vi "2_VisualizeModulePositioning2.vi"(0 "Placement Monitor":T6(plugin-control), 1 "Calibrated positions of fiducials [mm]":dbl[][](array[numeric])=[[-675.4228165149058, -196.82430550413875, -11.55], [-579.8428201474238, -196.8506568257386, -11.55], [-579.816468825824, -101.27066045825673, -11.55], [-675.3964651933059, -101.24430913665685, -11.55], [-577.422820239396, -196.8513240176017, -11.55], [-481.84282387191405, -196.87767533920157, -11.55], [-481.8164725503142, -101.29767897171968, -11.55], [-577.396468917796, -101.2713276501198, -11.55], [-479.42282396388623, -196.87834253106465, -11.55], [-383.8428275964043, -196.90469385266454, -11.55], [-383.81647627480436, -101.32469748518264, -11.55], [-479.3964726422863, -101.29834616358275, -11.55], [-381.42282768837646, -196.90536104452758, -11.55], [-285.8428313208945, -196.93171236612747, -11.55], [-285.8164799992946, -101.35171599864559, -11.55], [-381.39647636677654, -101.3253646770457, -11.55], [-283.4228314128667, -196.93237955799054, -11.55], [-187.84283504538473, -196.95873087959043, -11.55], [-187.8164837237848, -101.37873451210854, -11.55], [-283.39648009126677, -101.35238319050865, -11.55], [-185.42283513735697, -196.9593980714535, -11.55], [-89.84283876987502, -196.98574939305337, -11.55], [-89.81648744827521, -101.40575302557149, -11.55], [-185.39648381575705, -101.3794017039716, -11.55], [-87.42283886184703, -196.98641658491644, -11.55], [8.157157505634814, -197.01276790651633, -11.55], [8.183508827234618, -101.43277153903443, -11.55], [-87.39648754024722, -101.40642021743454, -11.55], [10.57715741366269, -197.01343509837938, -11.55], [106.15715378114453, -197.0397864199793, -11.55], [106.18350510274433, -101.45979005249738, -11.55], [10.603508735262494, -101.4334387308975, -11.55], [108.57715368917252, -197.04045361184234, -11.55], [204.15715005665436, -197.06680493344223, -11.55], [204.18350137825416, -101.48680856596033, -11.55], [108.60350501077232, -101.46045724436046, -11.55], [206.57714996468223, -197.0674721253053, -11.55], [302.1571463321641, -197.09382344690516, -11.55], [302.1834976537639, -101.5138270794233, -11.55], [206.60350128628204, -101.4874757578234, -11.55], [304.57714624019206, -197.09449063876826, -11.55], [400.1571426076739, -197.12084196036813, -11.55], [400.1834939292737, -101.54084559288623, -11.55], [304.60349756179187, -101.51449427128635, -11.55], [402.5771425157018, -197.1215091522312, -11.55], [498.15713888318373, -197.1478604738311, -11.55], [498.18349020478354, -101.56786410634919, -11.55], [402.6034938373016, -101.5415127847493, -11.55], [500.5771387912116, -197.14852766569413, -11.55], [596.1571351586933, -197.17487898729405, -11.55], [596.1834864802931, -101.59488261981214, -11.55], [500.6034901128114, -101.56853129821225, -11.55]], 2 "XYZ .NET Refnum in":refnum<k24>, 3 "Axis Speeds":T10={"X [mm/s]"=25.0, "Y [mm/s]"=25.0, "Z [mm/s]"=25.0}, 4 "Module fiducial marker":T7, 5 "N modules":i32=13, 6 "Sensor Pattern":T8(ring)=enum."ATLAS12", 7 "error in (no error)":errorcluster, 8 "Templates path":path=path "C:/Users/Aerotech/Documents/BNL_ThermomechanicalStave", 9 "Calibration [um/pix]":dbl=1.58, 10 "Current Build Phase":refnum<vi>, 12 "Module #":refnum<vi>, 13 "Placement tolerance [um]":dbl=25.0, 14 "Tape Type":T4=enum."Left stereo", 16 "Module Report":refnum<vi>, 17 "Base notes":string, 18 "Reports path":path=path "C:/Users/Aerotech/cernbox/BNL/Stave Assembly Records/2017-05-10") -> (22 "XYZ .NET Refnum out":refnum<k24>, 27 "error out":errorcluster)   [LabVIEW 2016]
uses:
  Utils/Enum_TypeDefinitions/Enum_TypeDef_FidMarkers.ctl
  C:/Users/Aerotech/Documents/BNL_ThermomechanicalStave/AerotechLibraries/Bin/Aerotech.A3200.dll
  AerotechLibraries/Bin/Aerotech.A3200.dll
  Utils/Enum_TypeDefinitions/Enum_TypeDef_CornerSelection.ctl
  Utils/Enum_TypeDefinitions/Enum_TypeDef_TapeType.ctl
panel:
  in  "Exit Module Placement":bool
  in  "Exit to survey or glue":bool
  out "Current task:":string
  in  "Tab Control: Positioning and Surveys":T1(tab)
  out "Offset interpreter":T2
  in  "User Report: Current Module":T3
  out "X offset [um]":sgl
  out "Y offset [um]":sgl
  in  "Module corner loop stop":bool
  in  "User notes":string="Type your note here...."
  out "Module # str":string
  in  "Assembly step":string(combo)
  in  "Calibrate distance?":bool=TRUE
  in  "Send XYZ stage beyond EOS":bool
  in  "Work on Corner...":T5=enum."[Exit]"
  in  "Work on Module #...":i32
  in  "Tab Control":enum32{"Fiducial marker", "Error reporting"}(tab)
  out "Fiducial Template":T6(plugin-control)
  out "Mark string":string
  out "Current Stage Position":T9
  out "Module Progress Report":T11(array[cluster])
  # "VISUALIZE MODULE PLACEMENT Brandeis University - Brookhaven National Laboratory * ATLAS Phase II Inner Tracker Upgrade"
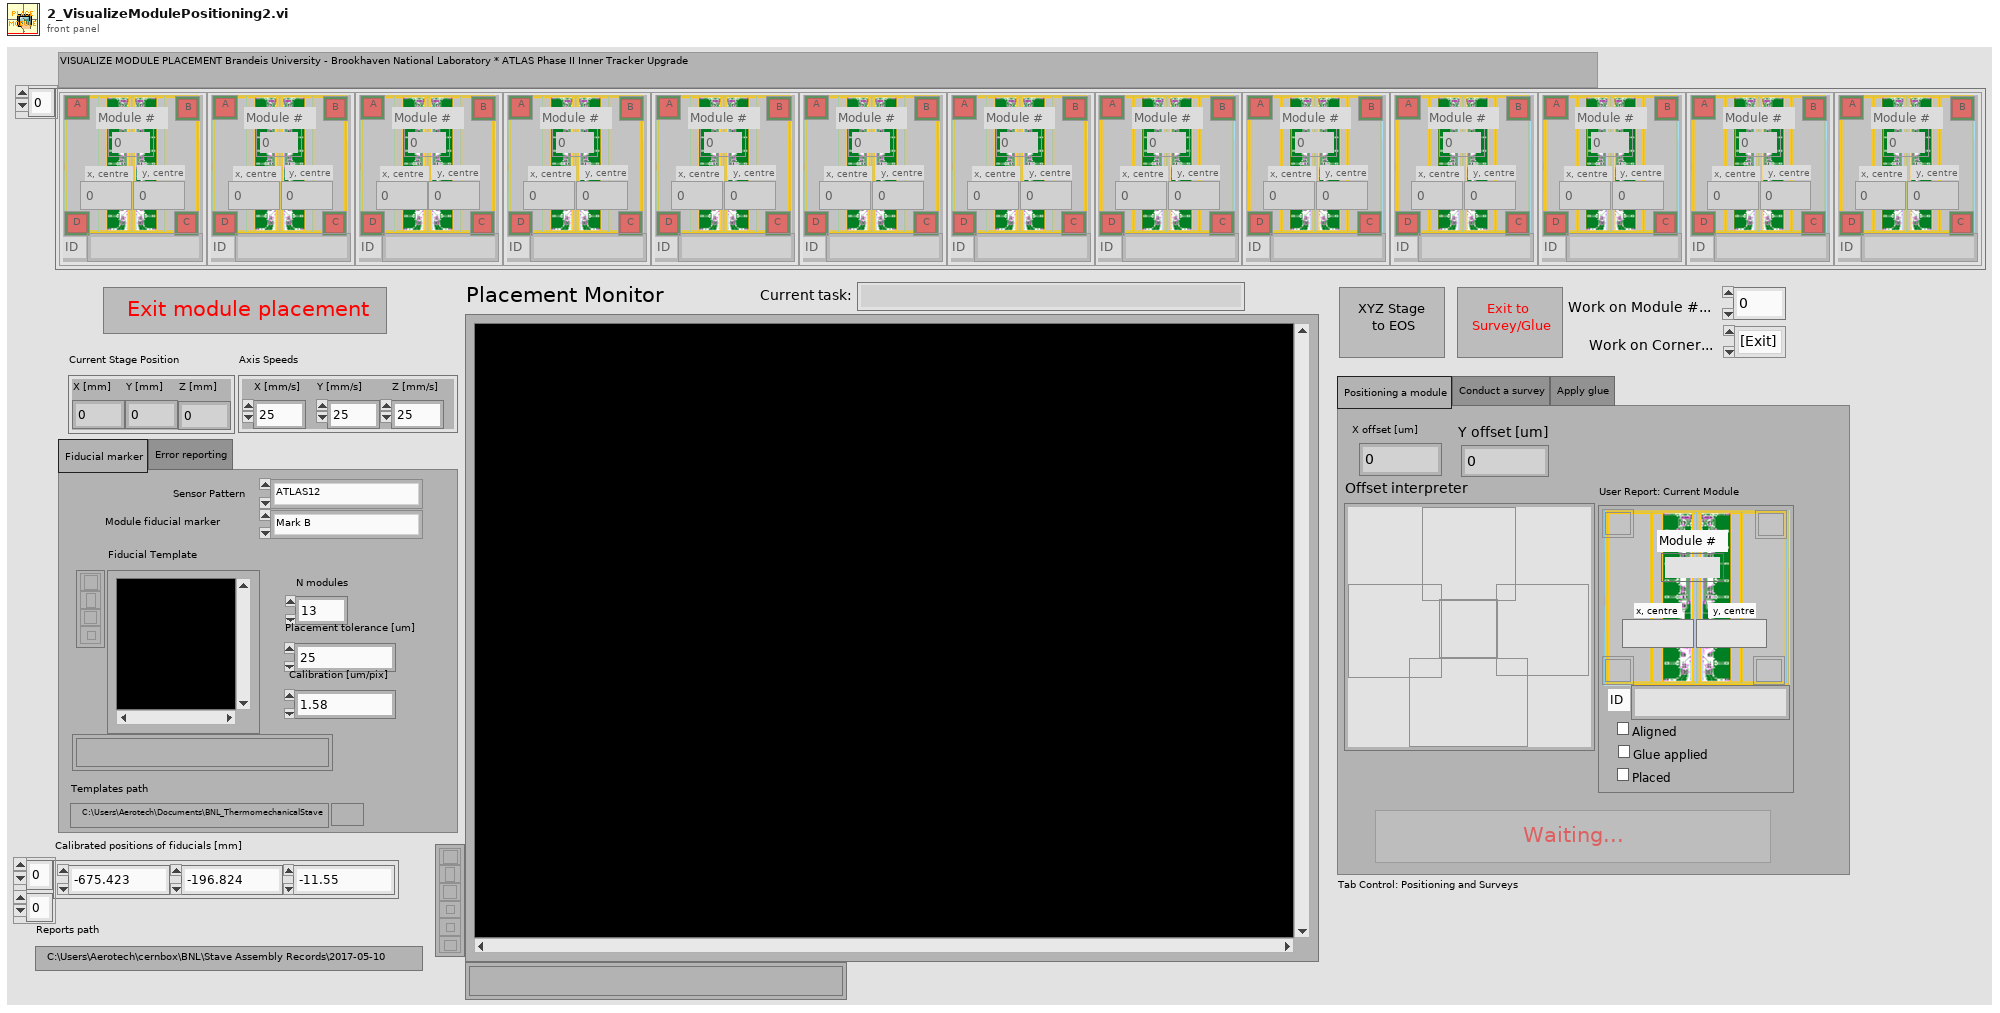
[diagram p1: front panel]
types:
  T1 = enum32{"Positioning a module", "Conduct a survey", "Apply glue"}
  T2 = cluster{"Offset Interpreter - Right":bool, "Offset Interpreter - forward":bool, "Offset Interpreter - backward":bool, "Offset Interpreter - Left":bool, "Placement Confirmation":bool}
  T3 = cluster{"B":bool, "A":bool, "D":bool, "C":bool, "ID":string, "Module #":i32, "x, centre":dbl, "y, centre":dbl, "Aligned":bool, "Glue applied":bool, "Placed":bool}
  T4 = typedef "Enum_TypeDef_TapeType.ctl" = enum16{"Right stereo", "Left stereo", "Stereo (Sutcliffe NP49-01-100 01-Mar-16)", "Axial (Sutcliffe NP49-01-100 01-Mar-16)"}
  T5 = typedef "Enum_TypeDef_CornerSelection.ctl" = enum16{"A", "B", "C", "D", "[Exit]"}
  T6 = typedef "IMAQ Image.ctl" = refnum<image>
  T7 = typedef "Enum_TypeDef_FidMarkers.ctl" = enum16{"Mark B", "Mark C", "Strip Corner", "Mark I (Slim/17)", "Mark E (Slim/17)", "Mark F (Slim/17)", "Mark G (Slim/17)", "Mark A (12)", "KaptonSpacers"}
  T8 = enum16{"ATLAS07", "ATLAS12", "ATLAS12Slim", "ATLAS17LS"}
  T9 = cluster{"X [mm]":dbl, "Y [mm]":dbl, "Z [mm]":dbl}
  T10 = cluster{"X [mm/s]":dbl, "Y [mm/s]":dbl, "Z [mm/s]":dbl}
  T11 = cluster{"B":bool, "A":bool, "D":bool, "C":bool, "ID":string, "Module #":i32, "x, centre":dbl, "y, centre":dbl, "Aligned":bool, "Glue applied":bool, "Placed":bool}[]
  T12 = enum8{"Enabled", "Disabled", "Disabled and Grayed Out"}
  T13 = enum16{"Left Button", "Center Button", "Right Button", "Window Close"}
  T14 = cluster{"Final X":dbl, "Final Y":dbl, "Final Z":dbl}
  T15 = cluster{"ID":string, "Mark string":string, "Assembly step":string, "User notes":string, string, "Corner surveyed position":dbl[]}
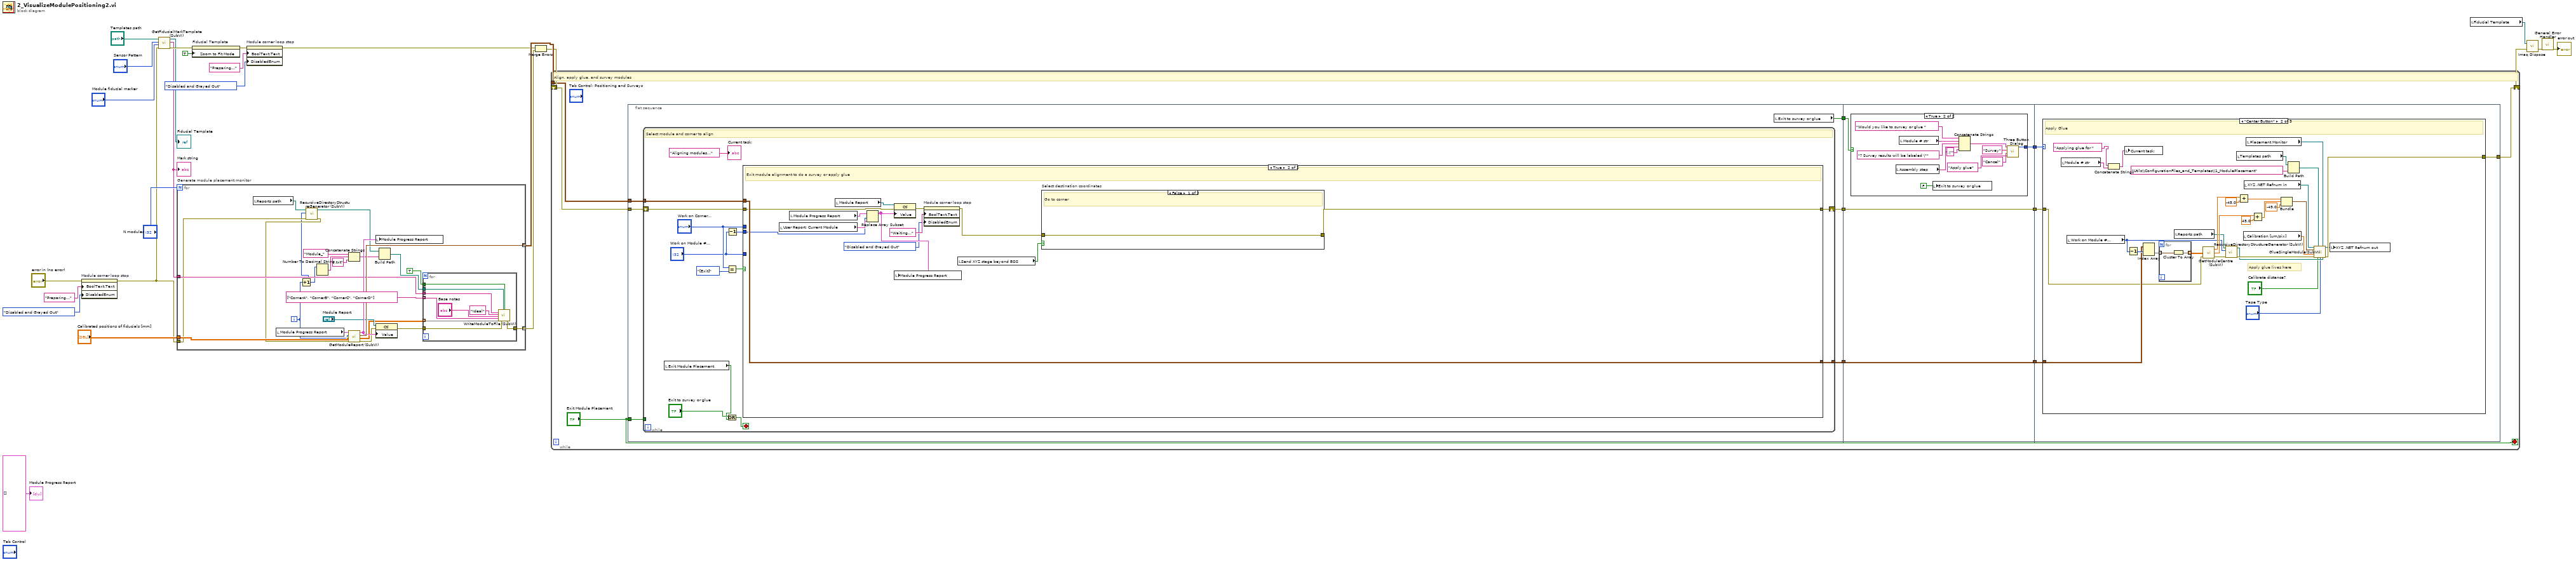
[diagram p0: block diagram]
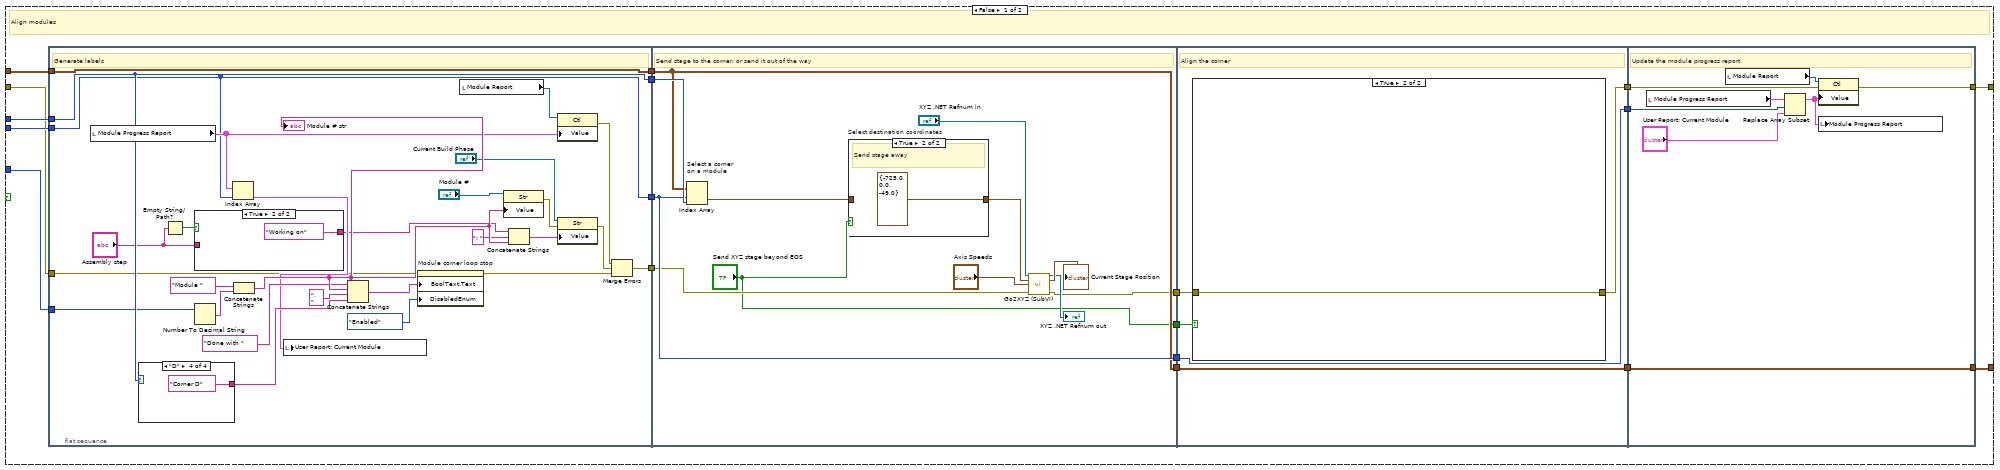
[diagram p2: hidden frame]
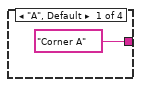
[diagram p4: hidden frame]
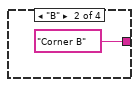
[diagram p5: hidden frame]
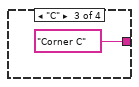
[diagram p6: hidden frame]
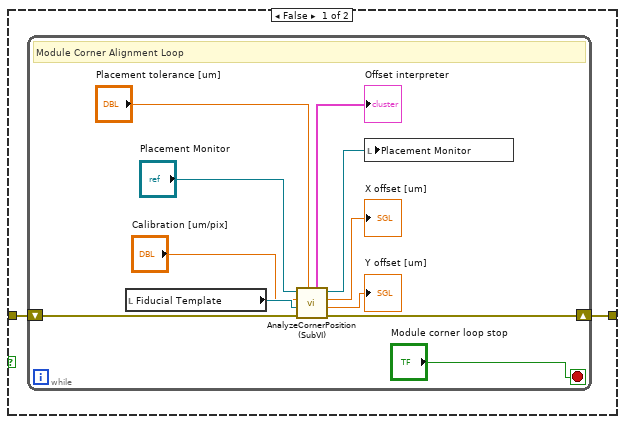
[diagram p8: hidden frame]
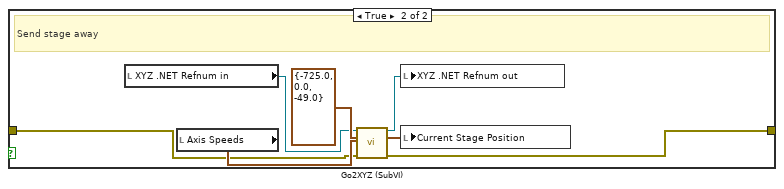
[diagram p9: hidden frame]
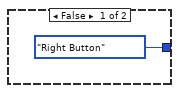
[diagram p10: hidden frame]
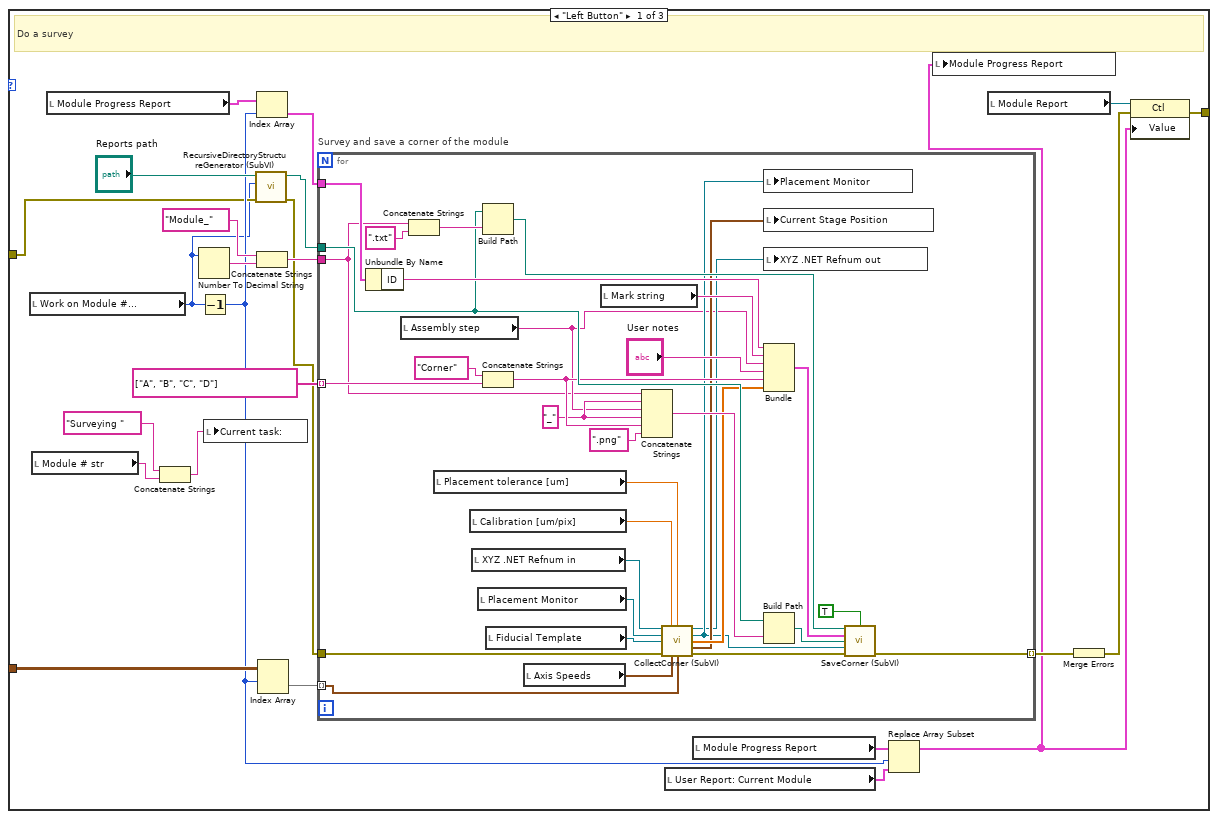
[diagram p11: hidden frame]
diagram:
  n1 = property on="Module corner loop stop" class="Bool"(error in="error in (no error)", "BoolText.Text"="Preparing..." ("Boolean Text.Text"), "DisabledEnum"=T12."Disabled and Grayed Out" ("Disabled")) -> (error out=w12:errorcluster)  [unwired: 1 in, 1 out]
  n2 = call "GetFiducialMarkTemplate (SubVI).vi"("error in (no error)"=w12, "Module fiducial marker"="Module fiducial marker", "Sensor Pattern"="Sensor Pattern", "Templates path"="Templates path") -> ("error out"=w16:errorcluster, "Mark string"=w2:string, "Template out"=→"Fiducial Template":T6)  [unwired: 5 in]
  "Mark string" <- w2
  n3 = for "Generate module placement monitor" {
    N: "N modules" -> [_]
    tunnel: "Calibrated positions of fiducials [mm]" -> [w48]
    tunnel: [w47] -> w9 mode=indexing
    tunnel: w12 -> [w28]
    tunnel: [w36] -> w1 mode=indexing
    tunnel: w2 -> [w32]
    i -> [w31]
    n4 = local read "Reports path"() -> (w30:path)
    n5 = local read "Module Progress Report"() -> (w43:T11)
    n6 = Increment(x=w31) -> (x+1=w26:i32)
    n7 = call "RecursiveDirectoryStructureGenerator (SubVI).vi"("error in (no error)"=w28, "Folder index"=w26, "Host directory"=w30) -> ("error out"=w27:errorcluster, "Nth subfolder in host directory"=w29:path)  [unwired: 7 in]
    n8 = Number To Decimal String(number=w26) -> (decimal integer string=w41:string)  [unwired: 1 in]
    n9 = Concatenate Strings("Module_" ("string"), w41, ".txt" ("string")) -> (w39:string)
    n10 = call "GetModuleReport (SubVI).vi"("error in (no error)"=w27, "Calibrated positions of fiducials [mm]"=w48, "ith Module"=w31, "Module Progress Report in"=w43) -> ("error out"=w45:errorcluster, "MyCorners"=w37:dbl[][], "Array of ith module cluster fiducial mark positions"=w47:cluster{"X":dbl, "Y":dbl, "Z":dbl}[], "Module Progress Report out"=w46:T11)  [unwired: 4 in]
    n11 = local write "Module Progress Report"(w46) -> ()
    n12 = property class="Ctl"(reference="Module Report", error in=w45, "Value"=w46) -> (error out=w35:errorcluster)  [unwired: 1 out]
    n13 = Build Path(base path=w29, name or relative path=w39) -> (appended path=w33:path)
    n14 = for {
      tunnel: string[] ["CornerA", "CornerB", "CornerC", "CornerD"] -> [w57] mode=indexing
      tunnel: w37 -> [w56] mode=indexing
      tunnel: [w55] -> w36
      tunnel: w35 -> [w54]
      tunnel: TRUE ("Write to file") -> [w53]
      tunnel: w33 -> [w52]
      tunnel: w32 -> [w51]
      n15 = call "WriteModuleToFile (SubVI).vi"("Mark used for tracking"=w51, "Assembly step"="Ideal", "User notes"="Base notes", "Current corner"=w57, "Fiducial Mark Position"=w56, "error in (no error)"=w54, "Module reports file path"=w52, "Write to file"=w53) -> ("error out"=w55:errorcluster)  [unwired: 11 in]
    }
  }
  n16 = property on="Fiducial Template" class="ImageControl"(error in=w16, "Zoom to Fit Mode"=TRUE) -> (error out=w8:errorcluster)  [unwired: 1 in, 1 out]
  n17 = property on="Module corner loop stop" class="Bool"(error in=w8, "BoolText.Text"="Preparing..." ("Boolean Text.Text"), "DisabledEnum"=T12."Disabled and Grayed Out" ("Disabled")) -> (error out=w3:errorcluster)  [unwired: 1 in, 1 out]
  n18 = Merge Errors(w3, w1) -> (w5:errorcluster)
  n19 = while {
    tunnel: w9 -> [w66]
    shift-right: [w62] -> w4
    shift-left: w5 -> [w65]
    stop <- "Exit Module Placement" stop-if-true
    # "Align, apply glue, and survey modules"
    n20 = flat-sequence {
      tunnel: w66 -> [w73]
      tunnel: w65 -> [w71]
      tunnel: [w72] -> w63
      tunnel: [w70] -> w61
      tunnel: "Exit Module Placement" -> [w69]
      tunnel: [w68] -> w58
      tunnel: [w204] -> w67
      tunnel: [w203] -> w64
      tunnel: w63 -> [w203]
      tunnel: w61 -> [w202]
      tunnel: [w202] -> w60
      tunnel: w58 -> [w201]
      tunnel: w67 -> [w220]
      tunnel: w64 -> [w219]
      tunnel: [w218] -> w62
      tunnel: w60 -> [w217]
      frame #0 {
        n21 = while {
          tunnel: w73 -> [w81]
          tunnel: [w80] -> w72
          shift-right: [w78] -> w70
          shift-left: w71 -> [w77]
          tunnel: w69 -> [_]
          stop <- w75 stop-if-true
          # "Select module and corner to align"
          n22 = local read "Exit Module Placement"() -> (w74:bool)
          n23 = Equal?(x="Work on Corner...", y=enum16{"A", "B", "C", "D", "[Exit]"}."[Exit]") -> (x = y?=w84:bool)
          n24 = Or(x="Exit to survey or glue", y=w74) -> (x .or. y?=w75:bool)
          n25 = Decrement(x="Work on Module #...") -> (x-1=w82:i32)
          n26 = case shown="True" w84 {
            tunnel: "Work on Corner..." -> [w104 _]
            tunnel: w82 -> [w102 w187]
            tunnel: w81 -> [w100 w188]
            tunnel: [w94 w188] -> w80
            tunnel: "Work on Module #..." -> [w93 _]
            tunnel: w77 -> [w92 w183]
            tunnel: [w88 w180] -> w78
            frame False {
              # "Align modules"
              n27 = flat-sequence {
                tunnel: w104 -> [w113]
                tunnel: [w113] -> w103
                tunnel: w102 -> [w111]
                tunnel: [w112] -> w101
                tunnel: w100 -> [w112]
                tunnel: [w111] -> w99
                tunnel: w93 -> [w110]
                tunnel: w92 -> [w109]
                tunnel: [w108] -> w91
                tunnel: w103 -> [w144]
                tunnel: w101 -> [w142]
                tunnel: w99 -> [w143]
                tunnel: [w143] -> w97
                tunnel: [w142] -> w95
                tunnel: w91 -> [w141]
                tunnel: [w140] -> w90
                tunnel: ["Send XYZ stage beyond EOS"] -> w87
                tunnel: [w157] -> w98
                tunnel: w97 -> [w157]
                tunnel: [w156] -> w96
                tunnel: w95 -> [w156]
                tunnel: w90 -> [w155]
                tunnel: [w154] -> w89
                tunnel: w87 -> [w153]
                tunnel: w98 -> [w175]
                tunnel: w96 -> [w174]
                tunnel: [w174] -> w94
                tunnel: w89 -> [w173]
                tunnel: [w172] -> w88
                frame #0 {
                  # "Generate labels"
                  n28 = local read "Module Progress Report"() -> (w115:T11)
                  n29 = case shown="\"D\"" w113 {
                    tunnel: ["Corner A" "Corner B" "Corner C" "Corner D"] -> w128
                    frame "A", Default {
                    }
                    frame "B" {
                    }
                    frame "C" {
                    }
                    frame "D" {
                    }
                  }
                  n30 = Empty String/Path?(string/path="Assembly step") -> (empty?=w107:bool)
                  n31 = case shown="True" w107 {
                    tunnel: [w133 "Working on" ("Assembly step")] -> w105
                    tunnel: "Assembly step" -> [w133 _]
                    frame False {
                    }
                    frame True {
                    }
                  }
                  n32 = Number To Decimal String(number=w110) -> (decimal integer string=w123:string)  [unwired: 1 in]
                  n33 = Index Array(array=w115, index=w111) -> (element=w114:T3)
                  n34 = Concatenate Strings("Module " ("string"), w123) -> (w129:string)
                  "Module # str" <- w129
                  n35 = local write "User Report: Current Module"(w114) -> ()
                  n36 = Concatenate Strings("Done with " ("string"), w129, ",  " ("string"), w128) -> (w127:string)
                  n37 = property on="Module corner loop stop" class="Bool"(error in=w109, "BoolText.Text"=w127, "DisabledEnum"=T12."Enabled" ("Disabled")) -> (error out=w132:errorcluster)  [unwired: 1 in, 1 out]
                  n38 = local read "Module Report"() -> (w116:refnum<vi>)
                  n39 = property class="Str"(reference="Module #", "Value"=w129) -> (error out=w120:errorcluster)  [unwired: 1 in, 1 out]
                  n40 = Concatenate Strings(w105, ": " ("string"), w129) -> (w121:string)
                  n41 = property class="Ctl"(reference=w116, "Value"=w115) -> (error out=w131:errorcluster)  [unwired: 1 in, 1 out]
                  n42 = property class="Str"(reference="Current Build Phase", error in=w120, "Value"=w121) -> (error out=w130:errorcluster)  [unwired: 1 out]
                  n43 = Merge Errors(w131, w130, w132) -> (w108:errorcluster)
                }
                frame #1 {
                  # "Send stage to the corner, or send it out of the way"
                  n44 = Index Array "Select a corner\non a module"(array=w142, index (row)=w143, index (col)=w144) -> (element=w145:cluster{"X":dbl, "Y":dbl, "Z":dbl})
                  n45 = case "Select destination coordinates" shown="True" "Send XYZ stage beyond EOS" {
                    tunnel: [w151 cluster{"X":dbl, "Y":dbl, "Z":dbl} {"X"=-725.0, "Y"=0.0, "Z"=-49.0}] -> w147
                    tunnel: w145 -> [w151 _]
                    frame False {
                      # "Go to corner"
                    }
                    frame True {
                      # "Send stage away"
                    }
                  }
                  n46 = call "Go2XYZ (SubVI).vi"(".NET Refnum in"="XYZ .NET Refnum in", "Go to Coordinates"=w147, "Axis Speeds"="Axis Speeds", "error in (no error)"=w141) -> (".NET Refnum out"=→"XYZ .NET Refnum out":refnum<k24>, "Final Position"=→"Current Stage Position":T14, "error out"=w140:errorcluster)  [unwired: 7 in, 2 out]
                }
                frame #2 {
                  # "Align the corner"
                  n47 = case shown="True" w153 {
                    tunnel: w155 -> [w159 w171]
                    tunnel: [w158 w171] -> w154
                    frame False {
                      n48 = while "Module Corner Placement Loop" {
                        shift-right: [w169] -> w158
                        shift-left: w159 -> [w160]
                        stop <- "Module corner loop stop" stop-if-true
                        # "Module Corner Alignment Loop"
                        n49 = local read "Fiducial Template"() -> (w168:T6)
                        n50 = call "AnalyzeCornerPosition (SubVI).vi"("Placement tolerance [um]"="Placement tolerance [um]", "error in (no error)"=w160, "Fiducial Template"=w168, "Calibration [um/pix]"="Calibration [um/pix]", "Refnum in"="Placement Monitor") -> ("error out"=w169:errorcluster, "Y offset [um]"=→"Y offset [um]":sgl, "X offset [um]"=→"X offset [um]":sgl, "Refnum out"=w167:T6, "Offset interpreter"=→"Offset interpreter":T2)  [unwired: 2 in]
                        n51 = local write "Placement Monitor"(w167) -> ()
                      }
                    }
                    frame True {
                    }
                  }
                }
                frame #3 {
                  # "Update the module progress report"
                  n52 = local read "Module Progress Report"() -> (w176:T11)
                  n53 = local read "Module Report"() -> (w179:refnum<vi>)
                  n54 = Replace Array Subset(array=w176, new element="User Report: Current Module", index=w175) -> (w177:T11)
                  n55 = property class="Ctl"(reference=w179, error in=w173, "Value"=w177) -> (error out=w172:errorcluster)  [unwired: 1 out]
                  n56 = local write "Module Progress Report"(w177) -> ()
                }
              }
            }
            frame True {
              # "Exit module alignment to do a survey or apply glue"
              n57 = local read "User Report: Current Module"() -> (w192:T3)
              n58 = local read "Module Progress Report"() -> (w189:T11)
              n59 = local read "Module Report"() -> (w191:refnum<vi>)
              n60 = Replace Array Subset(array=w189, new element=w192, index=w187) -> (w190:T11)
              n61 = property class="Ctl"(reference=w191, error in=w183, "Value"=w190) -> (error out=w184:errorcluster)  [unwired: 1 out]
              n62 = local write "Module Progress Report"(w190) -> ()
              n63 = property on="Module corner loop stop" class="Bool"(error in=w184, "BoolText.Text"="Waiting..." ("Boolean Text.Text"), "DisabledEnum"=T12."Disabled and Grayed Out" ("Disabled")) -> (error out=w181:errorcluster)  [unwired: 1 in, 1 out]
              n64 = local read "Send XYZ stage beyond EOS"() -> (w182:bool)
              n65 = case "Select destination coordinates" shown="False" w182 {
                tunnel: w181 -> [w193 w198]
                tunnel: [w193 w197] -> w180
                frame False {
                  # "Go to corner"
                }
                frame True {
                  # "Send stage away"
                  n66 = local read "XYZ .NET Refnum in"() -> (w195:refnum<k24>)
                  n67 = local read "Axis Speeds"() -> (w199:T10)
                  n68 = call "Go2XYZ (SubVI).vi"(".NET Refnum in"=w195, "Go to Coordinates"=cluster{"X":dbl, "Y":dbl, "Z":dbl} {"X"=-725.0, "Y"=0.0, "Z"=-49.0}, "Axis Speeds"=w199, "error in (no error)"=w198) -> (".NET Refnum out"=w196:refnum<k24>, "Final Position"=w194:T14, "error out"=w197:errorcluster)  [unwired: 7 in, 2 out]
                  n69 = local write "XYZ .NET Refnum out"(w196) -> ()
                  n70 = local write "Current Stage Position"(w194) -> ()
                }
              }
            }
          }
          "Current task:" <- "Aligning modules..." ("Prgm dialogue")
        }
        n71 = local read "Exit to survey or glue"() -> (w68:bool)
      }
      frame #1 {
        n72 = case shown="True" w201 {
          tunnel: [T13."Right Button" ("Which Button?") w213] -> w204
          frame False {
          }
          frame True {
            n73 = local read "Assembly step"() -> (w209:string)
            n74 = local read "Module # str"() -> (w212:string)
            n75 = local write "Exit to survey or glue"(FALSE ("Exit to survey or glue")) -> ()
            n76 = Concatenate Strings("Would you like to survey or glue " ("message"), w212, "? Survey results will be labeled \"" ("string"), w209, ".\"" ("string")) -> (w207:string)
            n77 = call <vilib>:"Three Button Dialog.vi"("Right Button Text (\"Cancel\")"="Cancel" ("Right Button Text (\"Cancel\")"), "Center Button Text (\"No\")"="Apply glue" ("Center Button Text (\"No\")"), "Left Button Text (\"Yes\")"="Survey" ("Left Button Text (\"Yes\")"), "message"=w207) -> ("Which Button?"=w213:T13)  [unwired: 7 in]
          }
        }
      }
      frame #2 {
        n78 = case shown="\"Center Button\"" w220 {
          tunnel: w219 -> [w242 w306 _]
          tunnel: [w230 w308 w311] -> w218
          tunnel: w217 -> [w226 w303 w311]
          frame "Left Button" {
            # "Do a survey"
            n79 = local read "Work on Module #..."() -> (w224:i32)
            n80 = local read "Module # str"() -> (w222:string)
            n81 = local read "Module Progress Report"() -> (w235:T11)
            n82 = Concatenate Strings("Surveying " ("Prgm dialogue"), w222) -> (w221:string)
            n83 = Number To Decimal String(number=w224) -> (decimal integer string=w243:string)  [unwired: 1 in]
            n84 = Decrement(x=w224) -> (x-1=w227:i32)
            n85 = local write "Current task:"(w221) -> ()
            n86 = call "RecursiveDirectoryStructureGenerator (SubVI).vi"("error in (no error)"=w226, "Folder index"=w224, "Host directory"="Reports path") -> ("error out"=w225:errorcluster, "Nth subfolder in host directory"=w229:path)  [unwired: 7 in]
            n87 = Index Array(array=w235, index=w227) -> (element=w233:T3)
            n88 = Concatenate Strings("Module_" ("string"), w243) -> (w231:string)
            n89 = Index Array(array=w242, index (row)=w227) -> (element=w244:cluster{"X":dbl, "Y":dbl, "Z":dbl}[])  [unwired: 1 in]
            n90 = for "Survey and save a corner of the module" {
              tunnel: w229 -> [w258]
              tunnel: [w273] -> w241 mode=indexing
              tunnel: w244 -> [w268] mode=indexing
              tunnel: string[] ["A", "B", "C", "D"] -> [w266] mode=indexing
              tunnel: w233 -> [w265]
              tunnel: w231 -> [w246]
              tunnel: w225 -> [w245]
              w248 = "_" ("string")
              n91 = Unbundle By Name(w265) -> ("ID"=w264:string)
              n92 = local read "Assembly step"() -> (w247:string)
              n93 = Concatenate Strings(w246, ".txt" ("string")) -> (w260:string)
              n94 = local read "Placement tolerance [um]"() -> (w271:dbl)
              n95 = local read "Calibration [um/pix]"() -> (w270:dbl)
              n96 = local read "XYZ .NET Refnum in"() -> (w277:refnum<k24>)
              n97 = local read "Placement Monitor"() -> (w272:T6)
              n98 = Build Path(base path=w258, name or relative path=w260) -> (appended path=w259:path)
              n99 = Concatenate Strings("Corner" ("string"), w266) -> (w256:string)
              n100 = local read "Fiducial Template"() -> (w276:T6)
              n101 = local read "Axis Speeds"() -> (w269:T10)
              n102 = local read "Mark string"() -> (w263:string)
              n103 = Concatenate Strings(w246, w248, w247, w248, w256, ".png" ("string")) -> (w255:string)
              n104 = call "CollectCorner (SubVI).vi"("XYZ .NET Refnum in"=w277, "Calibration [um/pix]"=w270, "Placement tolerance [um]"=w271, "Placement Monitor"=w272, "Fiducial Template"=w276, "error in (no error)"=w245, "Axis Speeds"=w269, "Corner Coordinates"=w268) -> ("XYZ .NET Refnum out"=w249:refnum<k24>, "Placement Monitor out"=w250:T6, "Corner surveyed position"=w253:dbl[], "XYZ Stage Final Position"=w251:T14, "error out"=w274:errorcluster)  [unwired: 3 in]
              n105 = local write "Placement Monitor"(w250) -> ()
              n106 = local write "Current Stage Position"(w251) -> ()
              n107 = local write "XYZ .NET Refnum out"(w249) -> ()
              n108 = Bundle("ID"=w264, "Mark string"=w263, "Assembly step"=w247, "User notes"="User notes", w256, "Corner surveyed position"=w253) -> (w252:T15)  [unwired: 1 in]
              n109 = Build Path(base path=w258, name or relative path=w255) -> (appended path=w254:path)
              n110 = call "SaveCorner (SubVI).vi"("Module record filename"=w259, "Write to file"=TRUE, "Data strings"=w252, "Module corner image filename"=w254, "Image of corner"=w250, "error in (no error)"=w274) -> ("error out"=w273:errorcluster)  [unwired: 9 in]
            }
            n111 = local read "User Report: Current Module"() -> (w240:T3)
            n112 = local read "Module Progress Report"() -> (w237:T11)
            n113 = Replace Array Subset(array=w237, new element=w240, index=w227) -> (w238:T11)
            n114 = local write "Module Progress Report"(w238) -> ()
            n115 = local read "Module Report"() -> (w239:refnum<vi>)
            n116 = Merge Errors(w241) -> (w236:errorcluster)
            n117 = property class="Ctl"(reference=w239, error in=w236, "Value"=w238) -> (error out=w230:errorcluster)  [unwired: 1 out]
          }
          frame "Center Button" {
            # "Apply glue lives here"
            # "Apply Glue"
            n118 = local read "Module # str"() -> (w281:string)
            n119 = local read "Work on Module #..."() -> (w289:i32)
            n120 = Concatenate Strings("Applying glue for " ("Prgm dialogue"), w281) -> (w280:string)
            n121 = local write "Current task:"(w280) -> ()
            n122 = Decrement(x=w289) -> (x-1=w307:i32)
            n123 = Index Array(array=w306, index (row)=w307) -> (element=w305:cluster{"X":dbl, "Y":dbl, "Z":dbl}[])  [unwired: 1 in]
            n124 = for {
              tunnel: w305 -> [w310] mode=indexing
              tunnel: [w309] -> w304 mode=indexing
              n125 = Cluster To Array(cluster=w310) -> (array=w309:dbl[])
            }
            n126 = local read "Reports path"() -> (w290:path)
            n127 = call "GetModuleCentre (SubVI).vi"("error in (no error)"=w303, "4x3 Array of Fiducial Coordinates"=w304) -> ("error out"=w288:errorcluster, "y, centre"=w299:dbl, "x, centre"=w302:dbl)  [unwired: 1 in]
            n128 = call "RecursiveDirectoryStructureGenerator (SubVI).vi"("error in (no error)"=w288, "Folder index"=w289, "Host directory"=w290) -> ("error out"=w287:errorcluster, "Nth subfolder in host directory"=w286:path)  [unwired: 7 in]
            n129 = local read "Templates path"() -> (w283:path)
            n130 = Add(x=w302, y=-45.0) -> (x+y=w297:dbl)
            n131 = local read "Calibration [um/pix]"() -> (w298:dbl)
            n132 = local read "XYZ .NET Refnum in"() -> (w293:refnum<k24>)
            n133 = local read "Placement Monitor"() -> (w291:T6)
            n134 = Add(x=w299, y=45.0) -> (x+y=w296:dbl)
            n135 = Bundle(w297, w296, "y"=-49.0) -> (w294:cluster{dbl, dbl, "y":dbl})  [unwired: 1 in]
            n136 = Build Path(base path=w283, name or relative path="Utils\\ConfigurationFiles_and_Templates\\1_ModulePlacement") -> (appended path=w282:path)
            n137 = call "GlueSingleModule(SubVI).vi"("XYZ Stage Control"=w293, "Template Path"=w282, "Image Feed"=w291, "Module corner coordinates"=w294, "um/pix resolution"=w298, "error in"=w287, "Calibrate distance?"="Calibrate distance?", "Tape Type"="Tape Type", "Path to save collected images"=w286) -> ("XYZ .NET Refnum out"=w292:refnum<k24>, "error out"=w308:errorcluster)  [unwired: 5 in]
            n138 = local write "XYZ .NET Refnum out"(w292) -> ()
          }
          frame "Right Button", Default {
            # "Do nothing -- go back to positioning modules"
            # "Do nothing (exit or return to module alignment)"
          }
        }
      }
    }
  }
  n139 = local read "Fiducial Template"() -> (w25:T6)
  n140 = call "Imaq Dispose"("Image"=w25, "error in (no error)"=w4) -> ("error out"=w24:errorcluster)  [unwired: 4 in]
  n141 = call <vilib>:"General Error Handler.vi"("error in (no error)"=w24) -> ("error out"=→"error out":errorcluster)  [unwired: 10 in, 4 out]
  "Module Progress Report" <- T11 [] ("Module Progress Report")
